vi "GAFM_Mockup.vi"() -> ()   [LabVIEW 2020]
panel:
  in  "Add to History":string
  out "History":string
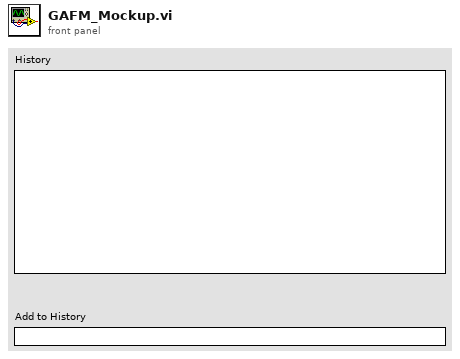
[diagram p1: front panel]
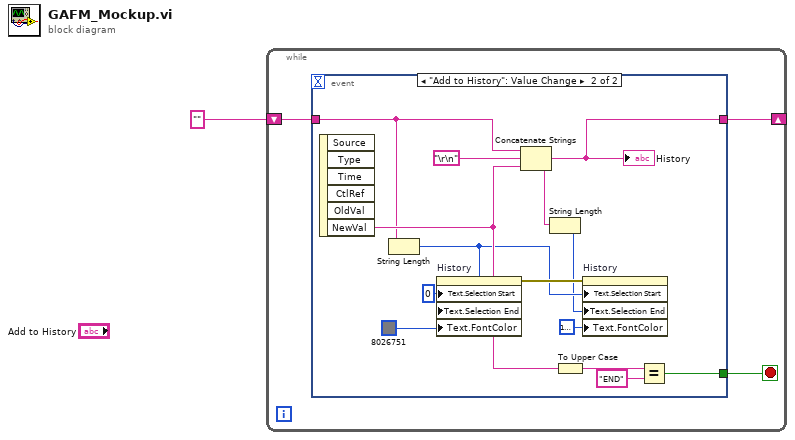
[diagram p0: block diagram]
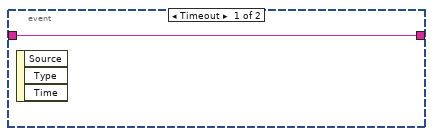
[diagram p2: hidden frame]
diagram:
  n1 = while {
    shift-right: [w2] -> _
    shift-left: "" -> [w3]
    stop <- w4 stop-if-true
    n2 = event shown="[1] \"Add to History\": Value Change" {
      selector: _ -> [_ _]
      dyn-events: _ -> [_ _]
      timeout: _ -> [_ _]
      tunnel: [_ w16] -> w4
      tunnel: w3 -> [w5 w12]
      tunnel: [w5 w8] -> w2
      event Timeout {
        n3 = event-data() -> ()  [unwired: 1 in, 3 out]
      }
      event "Add to History": Value Change {
        n4 = event-data() -> ("NewVal"=w14:string)  [unwired: 1 in, 5 out]
        n5 = String Length(string=w12) -> (length=w9:i32)
        n6 = property on="History" class="Str"("Text.Selection Start"=u32 0 ("Text.Selection:Start"), "Text.Selection End"=w9, "Text.FontColor"=u32 8026751 ("Text.Font:Color")) -> (error out=w10:errorcluster)  [unwired: 2 in, 1 out]
        n7 = Concatenate Strings(w12, "\r\n", w14) -> (w8:string)
        "History" <- w8
        n8 = String Length(string=w8) -> (length=w7:i32)
        n9 = To Upper Case(1:w14) -> (0:w18:string)
        n10 = property on="History" class="Str"(error in=w10, "Text.Selection Start"=w9, "Text.Selection End"=w7, "Text.FontColor"=u32 16777222 ("Text.Font:Color")) -> ()  [unwired: 1 in, 2 out]
        n11 = Equal?(x=w18, y="END") -> (x = y?=w16:bool)
      }
    }
  }
